vi "Get Spare Sensor Channels.vi"(10 "Existing":string[](array[string])) -> (0 "Deletable":string[](array[string]), 1 "Tasks":refnum<k21>[](array[refnum]), 2 "Spares":string[](array[string]))   [LabVIEW 2013]
uses:
  Data Access Objects/Metadata/Persistant DAO Actions.ctl
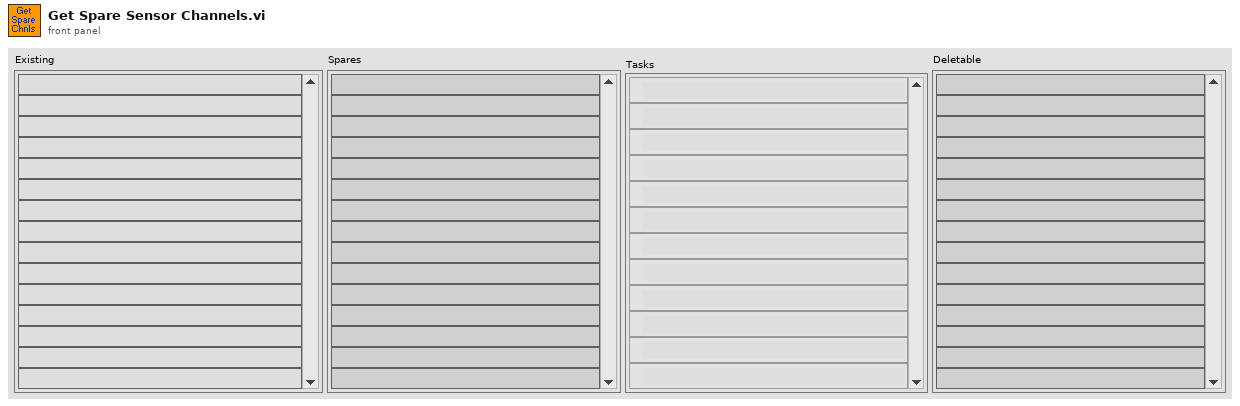
[diagram p1: front panel]
types:
  T1 = typedef "Persistant DAO Actions.ctl" = enum16{"Init", "Get", "Set", "Load", "Save"}
  T2 = typedef "DAQMx Tasks.ctl" = cluster{"LBCB1 Readings":refnum<k21>, "LBCB2 Readings":refnum<k21>, "LBCB1 Commands":refnum<k21>, "LBCB2 Commands":refnum<k21>, "Sensors":refnum<k21>[]}
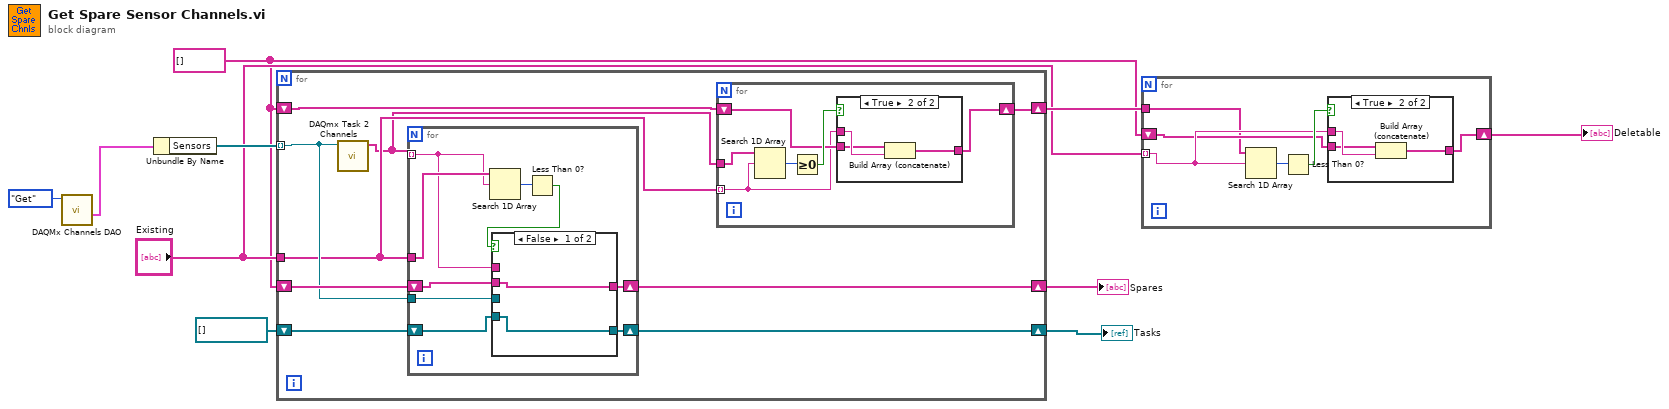
[diagram p0: block diagram]
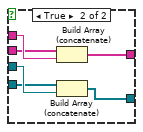
[diagram p4: hidden frame]
diagram:
  w2 = string[] []
  n1 = call "DAQMx Channels DAO.vi"("Actions"=Persistant_DAO_Actions."Get") -> ("Names Out"=w9:T2)  [unwired: 8 in, 2 out]
  n2 = Unbundle By Name(w9) -> ("Sensors"=w8:refnum<k21>[])
  n3 = for {
    tunnel: w8 -> [w17] mode=indexing
    tunnel: "Existing" -> [w14]
    shift-right: [w19] -> w7
    shift-left: w2 -> [w18]
    shift-right: [w16] -> w5
    shift-left: refnum<k21>[] [] -> [w15]
    shift-right: [w12] -> w4
    shift-left: w2 -> [w11]
    n4 = call "DAQmx Task 2 Channels.vi"("DAQmx Task Name"=w17) -> ("Channels Out"=w13:string[])  [unwired: 10 in]
    n5 = for {
      tunnel: w13 -> [w35] mode=indexing
      tunnel: w14 -> [w38]
      shift-right: [w34] -> w19
      shift-left: w18 -> [w33]
      tunnel: w17 -> [w32]
      shift-right: [w31] -> w16
      shift-left: w15 -> [w30]
      n6 = Search 1D Array(1D array=w38, element=w35) -> (index of element=w37:i32)  [unwired: 1 in]
      n7 = Less Than 0?(x=w37) -> (x < 0?=w36:bool)
      n8 = case shown="False" w36 {
        tunnel: w35 -> [_ w46]
        tunnel: [w40 w45] -> w34
        tunnel: w33 -> [w40 w44]
        tunnel: w32 -> [_ w43]
        tunnel: [w39 w42] -> w31
        tunnel: w30 -> [w39 w41]
        frame False {
        }
        frame True {
          n9 = Build Array (concatenate)(w44, w46) -> (w45:string[])
          n10 = Build Array (concatenate)(w41, w43) -> (w42:refnum<k21>[])
        }
      }
    }
    n11 = for {
      shift-right: [w21] -> w12
      shift-left: w11 -> [w22]
      tunnel: w14 -> [w20] mode=indexing
      tunnel: w13 -> [w24]
      n12 = Search 1D Array(1D array=w24, element=w20) -> (index of element=w25:i32)  [unwired: 1 in]
      n13 = Greater Or Equal To 0?(x=w25) -> (x >= 0?=w23:bool)
      n14 = case shown="True" w23 {
        tunnel: w20 -> [_ w29]
        tunnel: [w26 w28] -> w21
        tunnel: w22 -> [w26 w27]
        frame False {
        }
        frame True {
          n15 = Build Array (concatenate)(w27, w29) -> (w28:string[])
        }
      }
    }
  }
  "Spares" <- w7
  "Tasks" <- w5
  n16 = for {
    tunnel: w4 -> [w47]
    tunnel: "Existing" -> [w50] mode=indexing
    shift-right: [w48] -> w1
    shift-left: w2 -> [w49]
    n17 = Search 1D Array(1D array=w47, element=w50) -> (index of element=w51:i32)  [unwired: 1 in]
    n18 = Less Than 0?(x=w51) -> (x < 0?=w52:bool)
    n19 = case shown="True" w52 {
      tunnel: w50 -> [_ w56]
      tunnel: [w53 w55] -> w48
      tunnel: w49 -> [w53 w54]
      frame False {
      }
      frame True {
        n20 = Build Array (concatenate)(w54, w56) -> (w55:string[])
      }
    }
  }
  "Deletable" <- w1
